vi "Spectro_Init_Done.vi"(8 "error in (no error)":errorcluster, 10 "Variant":variant, 11 "Spectroscopy_Controller in":refnum<class "Spectroscopy_Controller.lvclass">) -> (0 "error out":errorcluster, 3 "Spectroscopy_Controller out":refnum<class "Spectroscopy_Controller.lvclass">)   [LabVIEW 2023, in "Spectroscopy_Controller.lvlib" / "Spectroscopy_Controller.lvclass"]
uses:
  Spectroscopy_Controller.lvclass
  Spectroscopy_Controller.lvclass/Spectroscopy_Controller.ctl
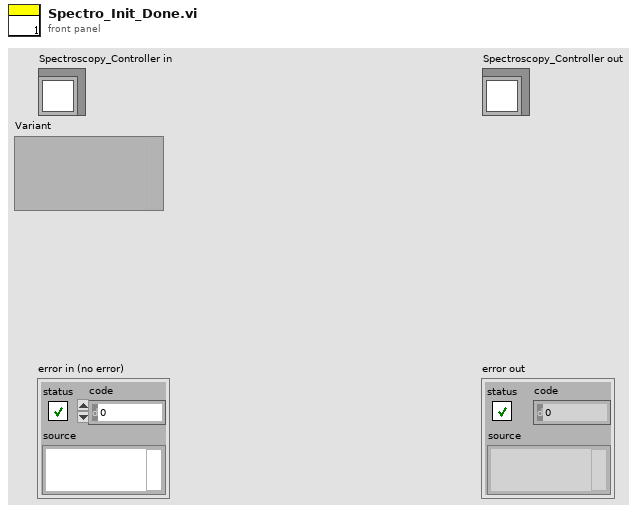
[diagram p1: front panel]
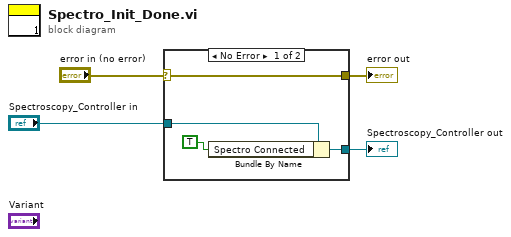
[diagram p0: block diagram]
diagram:
  n1 = case shown="No Error" "error in (no error)" {
    selector: "error in (no error)" -> [w8 w10]
    tunnel: [w8 w10] -> w3
    tunnel: [w5 w9] -> w1
    tunnel: "Spectroscopy_Controller in" -> [w6 w9]
    frame No Error {
      n2 = Bundle By Name(cluster=w6, "Spectro Connected"=TRUE ("SLM Connected")) -> (w5:refnum<class "Spectroscopy_Controller.lvclass">)
    }
    frame Error {
    }
  }
  "error out" <- w3
  "Spectroscopy_Controller out" <- w1
